vi "Helper-AssertControlValue.vi"() -> ()   [LabVIEW 2016, in "test_ValueSignal.lvlib"]
uses:
  test_ValueSignal.lvlib
panel:
  out "Product":dbl
  out "Result":bool
  in  "Stop":bool
  out "Number":i32
  in  "Reverse?":bool
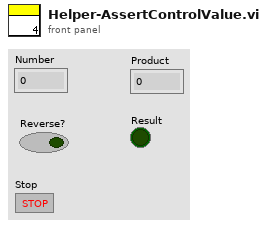
[diagram p1: front panel]
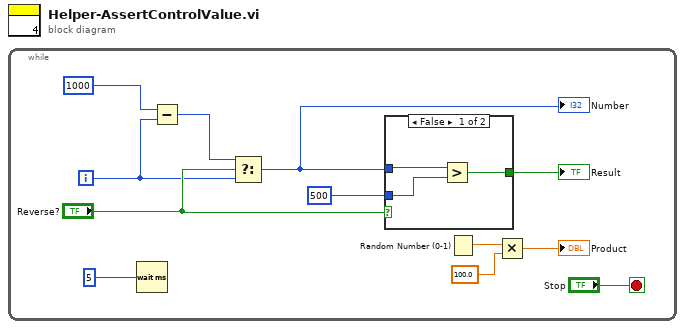
[diagram p0: block diagram]
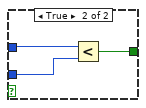
[diagram p2: hidden frame]
diagram:
  n1 = while {
    i -> [w6]
    stop <- "Stop" stop-if-true
    n2 = Wait (ms)(milliseconds to wait=u32 5) -> ()  [unwired: 1 out]
    n3 = Subtract(x=1000 ("y"), y=w6) -> (x-y=w7:i32)
    n4 = Select(t=w7, s="Reverse?", f=w6) -> (s? t:f=w9:i32)
    "Number" <- w9
    n5 = case shown="False" "Reverse?" {
      tunnel: 500 ("x") -> [w14 w18]
      tunnel: [w13 w17] -> w4
      tunnel: w9 -> [w15 w16]
      frame False {
        n6 = Greater?(x=w15, y=w14) -> (0:w13:bool)
      }
      frame True {
        n7 = Less?(x=w16, y=w18) -> (x < y?=w17:bool)
      }
    }
    "Result" <- w4
    n8 = Random Number (0-1)() -> (number: 0 to 1=w3:dbl)
    n9 = Multiply(x=w3, y=100.0) -> (x*y=→"Product":dbl)
  }
